vi "UICtrls_Disabled_Array.vi"(8 "error in":errorcluster, 9 "Disabled":T1(ring), 10 "Control Label":string[](array[string]), 11 "UI Ref cluster in":T2) -> (0 "error out":errorcluster, 3 "UI Ref cluster out":T2)   [LabVIEW 2025]
doc: "Enable\\Disable all Controls found"
uses:
  Controls/UI_Ref_Cluster.ctl
  <vilib>/Utility/Data Type/Type Definitions/Data Type.ctl
  UI_Manager.lvlib
  <vilib>/Utility/Data Type/NI_Data Type.lvlib
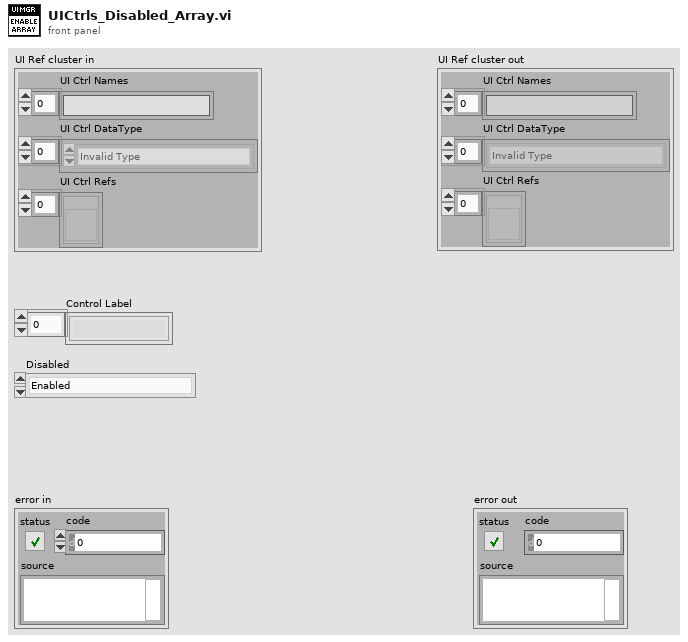
[diagram p1: front panel]
types:
  T1 = enum8{"Enabled", "Disabled", "Disabled and Grayed Out"}
  T2 = typedef "UI_Manager.lvlib/UI_Ref_Cluster.ctl" = cluster{"UI Ctrl Names":string[], "UI Ctrl DataType":T3[], "UI Ctrl Refs":refnum<vi>[]}
  T3 = typedef "NI_Data Type.lvlib/Data Type.ctl" = enum8{"Invalid Type", "Void", "I8", "I16", "I32", "I64", "U8", "U16", "U32", "U64", "Single Float", "Double Float", "Extended Float", "Single Complex", "Double Complex", "Extended Complex", "Enum U8", "Enum U16", "Enum U32", "Enum U64", "Single Float With Unit", "Double Float With Unit", "Extended Float With Unit", "Single Complex with Unit", "Double Complex with Unit", "Extended Complex with Unit", "Boolean", "String", "Path", "Picture", "Tag", "Array", "Cluster", "Variant", "LV Variant", "Waveform", "Timestamp", "Digital Waveform", "Digital Data", "ExpressData", "Refnum", "External Data", "VI", "Poly VI", "LabVIEW Class Instance", "Fixed Point", "Set Collection", "Map Collection"}
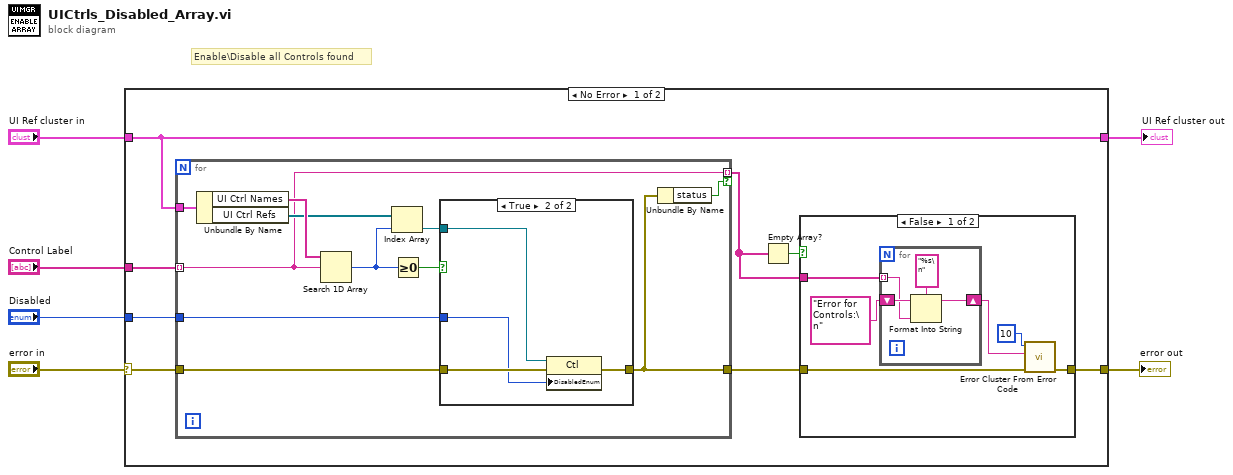
[diagram p0: block diagram]
diagram:
  # "Enable\\Disable all Controls found"
  n1 = case shown="No Error" "error in" {
    selector: "error in" -> [w13 w43]
    tunnel: [w10 w43] -> w6
    tunnel: "Control Label" -> [w14 _]
    tunnel: [w12 w42] -> w3
    tunnel: "UI Ref cluster in" -> [w12 w42]
    tunnel: "Disabled" -> [w11 _]
    frame No Error {
      n2 = for {
        tunnel: w14 -> [w28] mode=indexing
        tunnel: w12 -> [w30]
        tunnel: w11 -> [w29]
        tunnel: w13 -> [w31]
        tunnel: [w27] -> w9
        tunnel: [w28] -> w7 mode=indexing if=w26
        n3 = Unbundle By Name(w30) -> ("UI Ctrl Names"=w36:string[], "UI Ctrl Refs"=w34:refnum<vi>[])
        n4 = Search 1D Array(1D array=w36, element=w28) -> (index of element=w33:i32)  [unwired: 1 in]
        n5 = Index Array(array=w34, index=w33) -> (element=w32:refnum<vi>)
        n6 = Greater Or Equal To 0?(x=w33) -> (x >= 0?=w35:bool)
        n7 = case shown="True" w35 {
          tunnel: w32 -> [_ w41]
          tunnel: w31 -> [w37 w39]
          tunnel: [w37 w40] -> w27
          tunnel: w29 -> [_ w38]
          frame False {
          }
          frame True {
            n8 = property class="Ctl"(reference=w41, error in=w39, "DisabledEnum"=w38) -> (error out=w40:errorcluster)  [unwired: 1 out]
          }
        }
        n9 = Unbundle By Name(w27) -> ("status"=w26:bool)
      }
      n10 = Empty Array?(array=w7) -> (empty?=w8:bool)
      n11 = case shown="False" w8 {
        tunnel: [w20 w25] -> w10
        tunnel: w9 -> [w19 w25]
        tunnel: w7 -> [w15 _]
        frame False {
          n12 = for {
            tunnel: w15 -> [w22] mode=indexing
            shift-right: [w24] -> w17
            shift-left: "Error for Controls:\n" -> [w23]
            n13 = Format Into String(format string="%s\n", initial string=w23, w22) -> (resulting string=w24:string)  [unwired: 1 in, 1 out]
          }
          n14 = call <vilib>:"Error Cluster From Error Code.vi"("error in (no error)"=w19, "error message (\"\")"=w17, "error code (0)"=10) -> ("error out"=w20:errorcluster)  [unwired: 6 in]
        }
        frame True {
        }
      }
    }
    frame Error {
    }
  }
  "error out" <- w6
  "UI Ref cluster out" <- w3
